vi "S4GUI.vi"(7 "Tab ObsEng":enum32{"Obs", "CCD modes", "Guider", "Eng"}(tab)) -> ()   [LabVIEW 2018] (continued)
            n2447 = call-dynamic "Read Stream.vi"("error in (no error)"=w4925, "Server in"=w4926) -> ("error out"=w4929:errorcluster, "Stream.lvclass"=w4932:refnum<class "Stream.lvclass">, "Server out"=w4930:refnum<class "Acquisition.lvclass">)  [unwired: 7 in]
            n2448 = disable-structure shown="Enabled" {
              disable-tunnel: w4932 -> [w4938 w4948]
              disable-tunnel: [w4937 w4948] -> w4931
              disable-tunnel: w4929 -> [w4935 w4947]
              disable-tunnel: [w4933 w4947] -> w4928
              frame Disabled {
                w4946 = FALSE ("Wait Until Done")
                n2449 = call-dynamic "Read comfile name1.vi"("error in (no error)"=w4935, "Stream in"=w4938) -> ("error out"=w4934:errorcluster, "comfile name1"=w4941:string, "Stream out"=w4936:refnum<class "Stream.lvclass">)  [unwired: 7 in]
                n2450 = call <vilib>:"Application Directory.vi"() -> ("Application Directory"=w4943:path)
                n2451 = Build Path(base path=w4943, name or relative path=w4941) -> (appended path=w4942:path)
                n2452 = Open VI Reference(vi path=w4942, error in (no error)=w4934) -> (vi reference=w4944:refnum<vi>, error out=w4945:errorcluster)  [unwired: 4 in]
                n2453 = invoke class="VI" method="Run VI"(reference=w4944, error in=w4945, "Wait until done"=w4946, "Auto Dispose Ref"=w4946) -> (reference out=w4940:refnum<vi>, error out=w4939:errorcluster)  [unwired: 1 in, 3 out]
                n2454 = call-dynamic "Write commfile ref1.vi"("error in (no error)"=w4939, "commfile ref1"=w4940, "Stream in"=w4936) -> ("error out"=w4933:errorcluster, "Stream out"=w4937:refnum<class "Stream.lvclass">)  [unwired: 7 in]
              }
              frame Enabled {
              }
            }
          }
        }
        n2455 = call-dynamic "Write Stream.vi"("error in (no error)"=w4898, "Stream.lvclass"=w4899, "Server in"=w4894) -> ("error out"=w4880:errorcluster, "Server out"=w4881:refnum<class "Acquisition.lvclass">)  [unwired: 7 in]
        n2456 = call-dynamic "Write enabled.vi"("error in (no error)"=w4880, "enabled"=w4877, "Server in"=w4881) -> ("error out"=w4878:errorcluster, "Server out"=w4879:refnum<class "Acquisition.lvclass">)  [unwired: 7 in]
        n2457 = call-dynamic "Write Channel.vi"("error in (no error)"=w4878, "Channel.lvclass"=w4882, "Acquisition in"=w4879) -> ("error out"=w4888:errorcluster, "Acquisition out"=w4887:refnum<class "Acquisition.lvclass">)  [unwired: 7 in]
        n2458 = call-dynamic "Write AcquisitionC.vi"("error in (no error)"=w4888, "Acquisition.lvclass"=w4887, "S4ACS_GUI in"=w4886) -> ("error out"=w4891:errorcluster, "S4ACS_GUI out"=w4892:refnum<class "S4GUI.lvclass">)  [unwired: 7 in]
      }
      event "CH4 on": Value Change {
        n2459 = event-data() -> ("NewVal"=w4954:bool)  [unwired: 1 in]
        n2460 = call-dynamic "Read AcquisitionD.vi"("error in (no error)"=w4972, "S4ACS_GUI in"=w4973) -> ("error out"=w4964:errorcluster, "Acquisition.lvclass"=w4969:refnum<class "Acquisition.lvclass">, "S4ACS_GUI out"=w4965:refnum<class "S4GUI.lvclass">)  [unwired: 7 in]
        n2461 = call-dynamic "Read Channel.vi"("error in (no error)"=w4964, "Acquisition in"=w4969) -> ("error out"=w4963:errorcluster, "Channel.lvclass"=w4958:refnum<class "Channel.lvclass">, "Acquisition out"=w4968:refnum<class "Acquisition.lvclass">)  [unwired: 7 in]
        n2462 = call-dynamic "Read Stream.vi"("error in (no error)"=w4963, "Server in"=w4968) -> ("error out"=w4956:errorcluster, "Stream.lvclass"=w4955:refnum<class "Stream.lvclass">, "Server out"=w4957:refnum<class "Acquisition.lvclass">)  [unwired: 7 in]
        n2463 = case shown="False" w4954 {
          selector: w4954 -> [w4974 w4996]
          tunnel: [w4980 w5000] -> w4950
          tunnel: w4955 -> [w4989 _]
          tunnel: [w4988 w5003] -> w4951
          tunnel: w4956 -> [w4975 w4997]
          tunnel: w4957 -> [w4976 w4998]
          tunnel: [w4976 w5002] -> w4952
          tunnel: w4958 -> [w4987 w4999]
          tunnel: [w4985 w4999] -> w4953
          tunnel: [w4974 w4996] -> w4949
          frame False {
            # "força FALSE nos parametros do CCD"
            n2464 = call-dynamic "Read Interface.vi"("error in (no error)"=w4975, "Channel in"=w4987) -> ("error out"=w4984:errorcluster, "Interface.lvclass"=w4978:refnum<class "Interface.lvclass">, "Channel out"=w4986:refnum<class "Channel.lvclass">)  [unwired: 7 in]
            n2465 = disable-structure shown="Disabled" {
              disable-tunnel: w4989 -> [w4993 w4995]
              disable-tunnel: [w4992 w4995] -> w4988
              disable-tunnel: [w4991 w4994] -> w4981
              disable-tunnel: w4975 -> [w4990 w4994]
              frame Disabled {
                n2466 = call-dynamic "End.vi"("error in (no error)"=w4990, "Stream in"=w4993) -> ("error out"=w4991:errorcluster, "Stream out"=w4992:refnum<class "Stream.lvclass">)  [unwired: 8 in]
              }
              frame Enabled {
              }
            }
            n2467 = call "Write Checked Params.vi"("error in (no error)"=w4984, "Checked Params"=T14 {"ACQUISITION_MODE"=FALSE, "TRIGGER_MODE"=FALSE, "READ_MODE"=FALSE, "PREAMP"=FALSE, "READOUT_RATE"=FALSE, "VERTICAL_SHIFT_SPEED"=FALSE, "EM_MODE"=FALSE, "EM_GAIN"=FALSE, "SHUTTER_MODE"=FALSE, "SHUTTER_TTL"=FALSE, "SHUTTER_OPENING_TIME"=FALSE, "SHUTTER_CLOSING_TIME"=FALSE, "VBIN"=FALSE, "HBIN"=FALSE, "INITIAL_LINE"=FALSE, "INITIAL_COLUMN"=FALSE, "FINAL_LINE"=FALSE, "FINAL_COLUMN"=FALSE, "FRAME_TRANSFER"=FALSE, "VERTICAL_CLOCK_VOLTAGE"=FALSE, "AD_CHANNEL"=FALSE}, "Interface in"=w4978) -> ("error out"=w4983:errorcluster, "Interface out"=w4977:refnum<class "Interface.lvclass">)  [unwired: 7 in]
            n2468 = call-dynamic "Write Interface.vi"("error in (no error)"=w4983, "Interface.lvclass"=w4977, "Channel in"=w4986) -> ("error out"=w4982:errorcluster, "Channel out"=w4985:refnum<class "Channel.lvclass">)  [unwired: 7 in]
            n2469 = Merge Errors(w4982, w4981) -> (w4980:errorcluster)
          }
          frame True {
            n2470 = call-dynamic "Read Stream.vi"("error in (no error)"=w4997, "Server in"=w4998) -> ("error out"=w5001:errorcluster, "Stream.lvclass"=w5004:refnum<class "Stream.lvclass">, "Server out"=w5002:refnum<class "Acquisition.lvclass">)  [unwired: 7 in]
            n2471 = disable-structure shown="Enabled" {
              disable-tunnel: w5004 -> [w5010 w5020]
              disable-tunnel: [w5009 w5020] -> w5003
              disable-tunnel: w5001 -> [w5007 w5019]
              disable-tunnel: [w5005 w5019] -> w5000
              frame Disabled {
                w5018 = FALSE ("Wait Until Done")
                n2472 = call-dynamic "Read comfile name1.vi"("error in (no error)"=w5007, "Stream in"=w5010) -> ("error out"=w5006:errorcluster, "comfile name1"=w5013:string, "Stream out"=w5008:refnum<class "Stream.lvclass">)  [unwired: 7 in]
                n2473 = call <vilib>:"Application Directory.vi"() -> ("Application Directory"=w5015:path)
                n2474 = Build Path(base path=w5015, name or relative path=w5013) -> (appended path=w5014:path)
                n2475 = Open VI Reference(vi path=w5014, error in (no error)=w5006) -> (vi reference=w5016:refnum<vi>, error out=w5017:errorcluster)  [unwired: 4 in]
                n2476 = invoke class="VI" method="Run VI"(reference=w5016, error in=w5017, "Wait until done"=w5018, "Auto Dispose Ref"=w5018) -> (reference out=w5012:refnum<vi>, error out=w5011:errorcluster)  [unwired: 1 in, 3 out]
                n2477 = call-dynamic "Write commfile ref1.vi"("error in (no error)"=w5011, "commfile ref1"=w5012, "Stream in"=w5008) -> ("error out"=w5005:errorcluster, "Stream out"=w5009:refnum<class "Stream.lvclass">)  [unwired: 7 in]
              }
              frame Enabled {
              }
            }
          }
        }
        n2478 = call-dynamic "Write Stream.vi"("error in (no error)"=w4950, "Stream.lvclass"=w4951, "Server in"=w4952) -> ("error out"=w4960:errorcluster, "Server out"=w4962:refnum<class "Acquisition.lvclass">)  [unwired: 7 in]
        n2479 = call-dynamic "Write enabled.vi"("error in (no error)"=w4960, "enabled"=w4949, "Server in"=w4962) -> ("error out"=w4959:errorcluster, "Server out"=w4961:refnum<class "Acquisition.lvclass">)  [unwired: 7 in]
        n2480 = call-dynamic "Write Channel.vi"("error in (no error)"=w4959, "Channel.lvclass"=w4953, "Acquisition in"=w4961) -> ("error out"=w4967:errorcluster, "Acquisition out"=w4966:refnum<class "Acquisition.lvclass">)  [unwired: 7 in]
        n2481 = call-dynamic "Write AcquisitionD.vi"("error in (no error)"=w4967, "Acquisition.lvclass"=w4966, "S4ACS_GUI in"=w4965) -> ("error out"=w4970:errorcluster, "S4ACS_GUI out"=w4971:refnum<class "S4GUI.lvclass">)  [unwired: 7 in]
      }
      event "Run WPROT": Value Change {
        n2482 = event-data() -> ("NewVal"=w5028:bool)  [unwired: 1 in]
        n2483 = case shown="True" w5028 {
          tunnel: [u32 0 ("Ciclos  WPROT") "Ciclos  WPROT"] -> w5027
          tunnel: w5024 -> [w5030 w5035]
          tunnel: [w5030 w5034] -> w5023
          tunnel: w5022 -> [w5029 w5033]
          tunnel: [w5029 w5032] -> w5021
          frame False {
          }
          frame True {
            n2484 = call-dynamic "Write Obs_state.vi"("error in (no error)"=w5033, "Obs_state"=u32 350, "S4ACS_GUI in"=w5035) -> ("error out"=w5032:errorcluster, "S4ACS_GUI out"=w5034:refnum<class "S4GUI.lvclass">)  [unwired: 7 in]
          }
        }
        n2485 = call-dynamic "Write cycles wprot.vi"("error in (no error)"=w5021, "cycles wprot"=w5027, "S4GUI in"=w5023) -> ("error out"=w5025:errorcluster, "S4GUI out"=w5026:refnum<class "S4GUI.lvclass">)  [unwired: 7 in]
      }
      event "Start SM": Value Change {
        n2486 = event-data() -> ()  [unwired: 1 in, 6 out]
        n2487 = call-dynamic "Read Obs_state.vi"("error in (no error)"=w5064, "S4ACS_GUI in"=w5065) -> ("error out"=w5051:errorcluster, "Obs_state"=w5062:u32, "S4ACS_GUI out"=w5053:refnum<class "S4GUI.lvclass">)  [unwired: 7 in]
        n2488 = call "Read Instrument.lvclass.vi"("error in (no error)"=w5051, "S4ACS_GUI in"=w5053) -> ("error out"=w5049:errorcluster, "Instrument.lvclass"=w5050:refnum<class "Instrument.lvclass">, "S4ACS_GUI out"=w5052:refnum<class "S4GUI.lvclass">)  [unwired: 7 in]
        n2489 = Not Equal?(x=w5062, y=u32 400) -> (x != y?=w5061:bool)
        n2490 = call-dynamic "Read mode.vi"("error in (no error)"=w5049, "Instrument in"=w5050) -> ("error out"=w5048:errorcluster, "mode"=w5047:bool)  [unwired: 7 in, 1 out]
        n2491 = case shown="True" w5061 {
          tunnel: w5052 -> [w5107 w5195]
          tunnel: w5048 -> [w5108 w5194]
          tunnel: [w5111 w5201] -> w5042
          tunnel: [w5110 w5202] -> w5041
          tunnel: w5058 -> [_ w5209]
          tunnel: w5057 -> [_ w5208]
          tunnel: w5056 -> [_ w5207]
          tunnel: w5055 -> [_ w5206]
          tunnel: w5054 -> [_ w5205]
          tunnel: w5047 -> [_ w5204]
          tunnel: w5046 -> [_ w5185]
          tunnel: w5045 -> [_ w5188]
          tunnel: w5044 -> [_ w5187]
          tunnel: w5043 -> [_ w5186]
          tunnel: ["RESUME SM CLICKED" ("User Event") "START SM" ("User Event")] -> w5038
          frame False {
            # "Obs_state=400 (PAUSED), envia RESUME e vai para Obs_state=500 \npara esperar envio do comando RESUME a todos os canais."
            n2492 = call-dynamic "Write Obs_state.vi"("error in (no error)"=w5108, "Obs_state"=500, "S4ACS_GUI in"=w5107) -> ("error out"=w5112:errorcluster, "S4ACS_GUI out"=w5113:refnum<class "S4GUI.lvclass">)  [unwired: 7 in]
            n2493 = call-dynamic "Read AcquisitionA.vi"("error in (no error)"=w5112, "S4ACS_GUI in"=w5113) -> ("error out"=w5099:errorcluster, "Acquisition.lvclass"=w5103:refnum<class "Acquisition.lvclass">, "S4ACS_GUI out"=w5123:refnum<class "S4GUI.lvclass">)  [unwired: 7 in]
            n2494 = call-dynamic "Read enabled.vi"("error in (no error)"=w5099, "Server in"=w5103) -> ("error out"=w5101:errorcluster, "enabled"=w5100:bool, "Server out"=w5102:refnum<class "Acquisition.lvclass">)  [unwired: 7 in]
            n2495 = call-dynamic "Read Channel.vi"("error in (no error)"=w5101, "Acquisition in"=w5102) -> ("error out"=w5104:errorcluster, "Channel.lvclass"=w5105:refnum<class "Channel.lvclass">, "Acquisition out"=w5122:refnum<class "Acquisition.lvclass">)  [unwired: 7 in]
            n2496 = case shown="True" w5100 {
              tunnel: w5122 -> [w5170 w5183]
              tunnel: [w5170 w5182] -> w5121
              tunnel: [w5169 w5179] -> w5120
              tunnel: w5105 -> [_ w5172]
              tunnel: w5104 -> [w5169 w5171]
              frame False {
              }
              frame True {
                n2497 = call-dynamic "Read State Machine.vi"("error in (no error)"=w5171, "Device in"=w5172) -> ("error out"=w5173:errorcluster, "State Machine.lvclass"=w5174:refnum<class "State Machine.lvclass">, "Device out"=w5178:refnum<class "Channel.lvclass">)  [unwired: 7 in]
                n2498 = call "Next State.vi"("error in (no error)"=w5173, "New_State"=96, "State Machine in"=w5174) -> ("error out"=w5175:errorcluster, "State Machine out"=w5177:refnum<class "State Machine.lvclass">)  [unwired: 7 in]
                n2499 = call-dynamic "Write State Machine.vi"("error in (no error)"=w5175, "State Machine.lvclass"=w5177, "Device in"=w5178) -> ("error out"=w5180:errorcluster, "Device out"=w5181:refnum<class "Channel.lvclass">)  [unwired: 7 in]
                n2500 = call-dynamic "Write Channel.vi"("error in (no error)"=w5180, "Channel.lvclass"=w5181, "Acquisition in"=w5183) -> ("error out"=w5179:errorcluster, "Acquisition out"=w5182:refnum<class "Acquisition.lvclass">)  [unwired: 7 in]
              }
            }
            n2501 = call-dynamic "Write AcquisitionA.vi"("error in (no error)"=w5120, "Acquisition.lvclass"=w5121, "S4ACS_GUI in"=w5123) -> ("error out"=w5119:errorcluster, "S4ACS_GUI out"=w5116:refnum<class "S4GUI.lvclass">)  [unwired: 7 in]
            n2502 = call "Read AcquisitionB.vi"("error in (no error)"=w5119, "S4ACS_GUI in"=w5116) -> ("error out"=w5090:errorcluster, "Acquisition.lvclass"=w5091:refnum<class "Acquisition.lvclass">, "S4ACS_GUI out"=w5092:refnum<class "S4GUI.lvclass">)  [unwired: 7 in]
            n2503 = call-dynamic "Read enabled.vi"("error in (no error)"=w5090, "Server in"=w5091) -> ("error out"=w5094:errorcluster, "enabled"=w5093:bool, "Server out"=w5095:refnum<class "Acquisition.lvclass">)  [unwired: 7 in]
            n2504 = call-dynamic "Read Channel.vi"("error in (no error)"=w5094, "Acquisition in"=w5095) -> ("error out"=w5096:errorcluster, "Channel.lvclass"=w5097:refnum<class "Channel.lvclass">, "Acquisition out"=w5098:refnum<class "Acquisition.lvclass">)  [unwired: 7 in]
            n2505 = case shown="True" w5093 {
              tunnel: w5098 -> [w5155 w5168]
              tunnel: [w5155 w5167] -> w5089
              tunnel: [w5154 w5164] -> w5088
              tunnel: w5097 -> [_ w5157]
              tunnel: w5096 -> [w5154 w5156]
              frame False {
              }
              frame True {
                n2506 = call-dynamic "Read State Machine.vi"("error in (no error)"=w5156, "Device in"=w5157) -> ("error out"=w5158:errorcluster, "State Machine.lvclass"=w5159:refnum<class "State Machine.lvclass">, "Device out"=w5163:refnum<class "Channel.lvclass">)  [unwired: 7 in]
                n2507 = call "Next State.vi"("error in (no error)"=w5158, "New_State"=96, "State Machine in"=w5159) -> ("error out"=w5160:errorcluster, "State Machine out"=w5162:refnum<class "State Machine.lvclass">)  [unwired: 7 in]
                n2508 = call-dynamic "Write State Machine.vi"("error in (no error)"=w5160, "State Machine.lvclass"=w5162, "Device in"=w5163) -> ("error out"=w5165:errorcluster, "Device out"=w5166:refnum<class "Channel.lvclass">)  [unwired: 7 in]
                n2509 = call-dynamic "Write Channel.vi"("error in (no error)"=w5165, "Channel.lvclass"=w5166, "Acquisition in"=w5168) -> ("error out"=w5164:errorcluster, "Acquisition out"=w5167:refnum<class "Acquisition.lvclass">)  [unwired: 7 in]
              }
            }
            n2510 = call "Write AcquisitionB.vi"("error in (no error)"=w5088, "Acquisition.lvclass"=w5089, "S4ACS_GUI in"=w5092) -> ("error out"=w5118:errorcluster, "S4ACS_GUI out"=w5115:refnum<class "S4GUI.lvclass">)  [unwired: 7 in]
            n2511 = call-dynamic "Read AcquisitionC.vi"("error in (no error)"=w5118, "S4ACS_GUI in"=w5115) -> ("error out"=w5078:errorcluster, "Acquisition.lvclass"=w5081:refnum<class "Acquisition.lvclass">, "S4ACS_GUI out"=w5080:refnum<class "S4GUI.lvclass">)  [unwired: 7 in]
            n2512 = call-dynamic "Read enabled.vi"("error in (no error)"=w5078, "Server in"=w5081) -> ("error out"=w5083:errorcluster, "enabled"=w5082:bool, "Server out"=w5084:refnum<class "Acquisition.lvclass">)  [unwired: 7 in]
            n2513 = call-dynamic "Read Channel.vi"("error in (no error)"=w5083, "Acquisition in"=w5084) -> ("error out"=w5085:errorcluster, "Channel.lvclass"=w5086:refnum<class "Channel.lvclass">, "Acquisition out"=w5087:refnum<class "Acquisition.lvclass">)  [unwired: 7 in]
            n2514 = case shown="True" w5082 {
              tunnel: w5087 -> [w5140 w5153]
              tunnel: [w5140 w5152] -> w5079
              tunnel: [w5139 w5149] -> w5077
              tunnel: w5086 -> [_ w5142]
              tunnel: w5085 -> [w5139 w5141]
              frame False {
              }
              frame True {
                n2515 = call-dynamic "Read State Machine.vi"("error in (no error)"=w5141, "Device in"=w5142) -> ("error out"=w5143:errorcluster, "State Machine.lvclass"=w5144:refnum<class "State Machine.lvclass">, "Device out"=w5148:refnum<class "Channel.lvclass">)  [unwired: 7 in]
                n2516 = call "Next State.vi"("error in (no error)"=w5143, "New_State"=96, "State Machine in"=w5144) -> ("error out"=w5145:errorcluster, "State Machine out"=w5147:refnum<class "State Machine.lvclass">)  [unwired: 7 in]
                n2517 = call-dynamic "Write State Machine.vi"("error in (no error)"=w5145, "State Machine.lvclass"=w5147, "Device in"=w5148) -> ("error out"=w5150:errorcluster, "Device out"=w5151:refnum<class "Channel.lvclass">)  [unwired: 7 in]
                n2518 = call-dynamic "Write Channel.vi"("error in (no error)"=w5150, "Channel.lvclass"=w5151, "Acquisition in"=w5153) -> ("error out"=w5149:errorcluster, "Acquisition out"=w5152:refnum<class "Acquisition.lvclass">)  [unwired: 7 in]
              }
            }
            n2519 = call-dynamic "Write AcquisitionC.vi"("error in (no error)"=w5077, "Acquisition.lvclass"=w5079, "S4ACS_GUI in"=w5080) -> ("error out"=w5117:errorcluster, "S4ACS_GUI out"=w5114:refnum<class "S4GUI.lvclass">)  [unwired: 7 in]
            n2520 = call-dynamic "Read AcquisitionD.vi"("error in (no error)"=w5117, "S4ACS_GUI in"=w5114) -> ("error out"=w5068:errorcluster, "Acquisition.lvclass"=w5069:refnum<class "Acquisition.lvclass">, "S4ACS_GUI out"=w5070:refnum<class "S4GUI.lvclass">)  [unwired: 7 in]
            n2521 = call-dynamic "Read enabled.vi"("error in (no error)"=w5068, "Server in"=w5069) -> ("error out"=w5072:errorcluster, "enabled"=w5071:bool, "Server out"=w5073:refnum<class "Acquisition.lvclass">)  [unwired: 7 in]
            n2522 = call-dynamic "Read Channel.vi"("error in (no error)"=w5072, "Acquisition in"=w5073) -> ("error out"=w5074:errorcluster, "Channel.lvclass"=w5075:refnum<class "Channel.lvclass">, "Acquisition out"=w5076:refnum<class "Acquisition.lvclass">)  [unwired: 7 in]
            n2523 = case shown="True" w5071 {
              tunnel: w5076 -> [w5125 w5138]
              tunnel: [w5125 w5137] -> w5067
              tunnel: [w5124 w5134] -> w5066
              tunnel: w5075 -> [_ w5127]
              tunnel: w5074 -> [w5124 w5126]
              frame False {
              }
              frame True {
                n2524 = call-dynamic "Read State Machine.vi"("error in (no error)"=w5126, "Device in"=w5127) -> ("error out"=w5128:errorcluster, "State Machine.lvclass"=w5129:refnum<class "State Machine.lvclass">, "Device out"=w5133:refnum<class "Channel.lvclass">)  [unwired: 7 in]
                n2525 = call "Next State.vi"("error in (no error)"=w5128, "New_State"=96, "State Machine in"=w5129) -> ("error out"=w5130:errorcluster, "State Machine out"=w5132:refnum<class "State Machine.lvclass">)  [unwired: 7 in]
                n2526 = call-dynamic "Write State Machine.vi"("error in (no error)"=w5130, "State Machine.lvclass"=w5132, "Device in"=w5133) -> ("error out"=w5135:errorcluster, "Device out"=w5136:refnum<class "Channel.lvclass">)  [unwired: 7 in]
                n2527 = call-dynamic "Write Channel.vi"("error in (no error)"=w5135, "Channel.lvclass"=w5136, "Acquisition in"=w5138) -> ("error out"=w5134:errorcluster, "Acquisition out"=w5137:refnum<class "Acquisition.lvclass">)  [unwired: 7 in]
              }
            }
            n2528 = call-dynamic "Write AcquisitionD.vi"("error in (no error)"=w5066, "Acquisition.lvclass"=w5067, "S4ACS_GUI in"=w5070) -> ("error out"=w5110:errorcluster, "S4ACS_GUI out"=w5111:refnum<class "S4GUI.lvclass">)  [unwired: 7 in]
          }
          frame True {
            # "vide S4GUI:\nHandleObservationSync.vi"
            # "aba atual em Tab Acq Type"
            n2529 = call "Read Instrument.lvclass.vi"("error in (no error)"=w5194, "S4ACS_GUI in"=w5195) -> ("error out"=w5197:errorcluster, "Instrument.lvclass"=w5199:refnum<class "Instrument.lvclass">, "S4ACS_GUI out"=w5192:refnum<class "S4GUI.lvclass">)  [unwired: 7 in]
            n2530 = call "Read WPROT.vi"("error in (no error)"=w5197, "Instrument in"=w5199) -> ("error out"=w5196:errorcluster, "Opt_Selector.lvclass"=w5198:refnum<class "Opt_Selector.lvclass">)  [unwired: 7 in, 1 out]
            n2531 = call-dynamic "Read sequencia.vi"("error in (no error)"=w5196, "Opt_Selector in"=w5198) -> ("error out"=w5191:errorcluster, "sequencia"=w5193:u16)  [unwired: 7 in, 1 out]
            n2532 = case shown="\"FOCUS\"" w5185 {
              tunnel: [u32 271 ("Obs_state") u32 251 ("Obs_state")] -> w5212
              tunnel: w5192 -> [w5233 w5236]
              tunnel: w5191 -> [w5223 w5235]
              tunnel: [w5231 w5236] -> w5190
              tunnel: [w5222 w5235] -> w5189
              tunnel: w5188 -> [w5230 _]
              tunnel: w5187 -> [w5229 _]
              tunnel: w5186 -> [w5228 _]
              frame "FOCUS" {
                n2533 = call-dynamic "Read TelFocus.lvclass.vi"("error in (no error)"=w5223, "S4GUI in"=w5233) -> ("error out"=w5225:errorcluster, "TelFocus.lvclass"=w5227:refnum<class "TelFocus.lvclass">, "S4GUI out"=w5232:refnum<class "S4GUI.lvclass">)  [unwired: 7 in]
                n2534 = call-dynamic "LoadParam.vi"("#steps"=w5228, "error in (no error)"=w5225, "step"=w5229, "init"=w5230, "TelFocus in"=w5227) -> ("error out"=w5224:errorcluster, "TelFocus out"=w5226:refnum<class "TelFocus.lvclass">)  [unwired: 5 in]
                n2535 = call-dynamic "Write TelFocus.lvclass.vi"("error in (no error)"=w5224, "TelFocus.lvclass"=w5226, "S4GUI in"=w5232) -> ("error out"=w5222:errorcluster, "S4GUI out"=w5231:refnum<class "S4GUI.lvclass">)  [unwired: 7 in]
              }
              frame Default {
              }
            }
            n2536 = case shown="Default" w5185 {
              tunnel: w5204 -> [_ w5218]
              tunnel: [u32 1 ("# Cycles") w5217] -> w5203
              tunnel: [u32 1 w5216] -> w5200
              tunnel: w5193 -> [_ w5215]
              frame "FOCUS" {
                # "Aba FOCUS: Para a sequencia de foco, sempre  #Cycles=1 e #Seqs=1"
              }
              frame Default {
                n2537 = case shown="False" w5218 {
                  tunnel: [0 w5221] -> w5216
                  tunnel: w5215 -> [_ w5220]
                  frame False {
                    # "OV 20230424: \n#SEQ agora armazena as\nposições da lâmina utilizadas.\nNa fotometria, #SEQ=0"
                    # "fotometria:"
                  }
                  frame True {
                    # "OV 20230424: \n#SEQ agora armazena as\nposições da lâmina utilizadas.\nNa polarimetria, #SEQ=WPROT.sequencia"
                    # "polarimetria:"
                    n2538 = To Unsigned Long Integer(number=w5220) -> (unsigned 32bit integer=w5221:u32)
                  }
                }
                n2539 = local read "# Cycles"() -> (w5217:u32)
              }
            }
            n2540 = call-dynamic "Write Obs_state.vi"("error in (no error)"=w5189, "Obs_state"=w5212, "S4ACS_GUI in"=w5190) -> ("error out"=w5211:errorcluster, "S4ACS_GUI out"=w5210:refnum<class "S4GUI.lvclass">)  [unwired: 7 in]
            n2541 = stacked-sequence {
              seq-local: [w5260 _ _ _] -> [_ w5332 _ _]
              seq-local: [w5259 _ _ _] -> [_ w5331 _ _]
              seq-local: [_ w5330 _ _] -> [_ _ w5383 _]
              seq-local: [_ w5329 _ _] -> [_ _ w5382 _]
              seq-local: [_ _ w5381 _] -> [_ _ _ w5434]
              seq-local: [_ _ w5380 _] -> [_ _ _ w5433]
              tunnel: w5211 -> [w5275 _ _ _]
              tunnel: w5210 -> [w5274 _ _ _]
              tunnel: [_ _ _ w5432] -> w5201
              tunnel: [_ _ _ w5431] -> w5202
              tunnel: w5209 -> [w5258 w5328 w5379 w5430]
              tunnel: w5208 -> [w5257 w5327 w5359 w5410]
              tunnel: w5207 -> [w5256 w5307 w5358 w5409]
              tunnel: w5206 -> [w5255 w5306 w5357 w5408]
              tunnel: w5205 -> [w5250 w5303 w5354 w5405]
              tunnel: w5203 -> [_ _ _ _]
              tunnel: w5200 -> [_ _ _ _]
              tunnel: w5185 -> [w5242 w5297 w5348 w5397]
              frame #0 {
                # "object"
                # "suffix"
                # "obsType"
                n2542 = local read "Exptime ch1"() -> (w5243:dbl)
                n2543 = call-dynamic "Read AcquisitionA.vi"("error in (no error)"=w5275, "S4ACS_GUI in"=w5274) -> ("error out"=w5273:errorcluster, "Acquisition.lvclass"=w5272:refnum<class "Acquisition.lvclass">, "S4ACS_GUI out"=w5263:refnum<class "S4GUI.lvclass">)  [unwired: 7 in]
                n2544 = call-dynamic "Read Channel.vi"("error in (no error)"=w5273, "Acquisition in"=w5272) -> ("error out"=w5270:errorcluster, "Channel.lvclass"=w5271:refnum<class "Channel.lvclass">, "Acquisition out"=w5262:refnum<class "Acquisition.lvclass">)  [unwired: 7 in]
                n2545 = call-dynamic "Read Interface.vi"("error in (no error)"=w5270, "Channel in"=w5271) -> ("error out"=w5281:errorcluster, "Interface.lvclass"=w5268:refnum<class "Interface.lvclass">, "Channel out"=w5269:refnum<class "Channel.lvclass">)  [unwired: 7 in]
                n2546 = call "Write Exposure Time.vi"("error in (no error)"=w5281, "Exposure Time"=w5243, "Interface in"=w5268) -> ("error out"=w5244:errorcluster, "Interface out"=w5247:refnum<class "Interface.lvclass">)  [unwired: 7 in]
                n2547 = case shown="Default" w5242 {
                  tunnel: w5247 -> [w5283 w5288]
                  tunnel: [w5283 w5287] -> w5246
                  tunnel: [w5282 w5286] -> w5245
                  tunnel: w5244 -> [w5282 w5285]
                  tunnel: w5243 -> [_ w5284]
                  frame "ZERO" {
                  }
                  frame Default {
                    n2548 = call-dynamic "Write prev ExpTime.vi"("error in (no error)"=w5285, "prev ExpTime"=w5284, "Interface in"=w5288) -> ("error out"=w5286:errorcluster, "Interface out"=w5287:refnum<class "Interface.lvclass">)  [unwired: 7 in]
                  }
                }
                n2549 = call-dynamic "Write Suffix.vi"("error in (no error)"=w5245, "Suffix"=w5258, "Interface in"=w5246) -> ("error out"=w5280:errorcluster, "Interface out"=w5267:refnum<class "Interface.lvclass">)  [unwired: 7 in]
                n2550 = call-dynamic "Write ObsType.vi"("error in (no error)"=w5280, "ObsType"=w5256, "Interface in"=w5267) -> ("error out"=w5279:errorcluster, "Interface out"=w5266:refnum<class "Interface.lvclass">)  [unwired: 7 in]
                n2551 = call-dynamic "Write Object.vi"("error in (no error)"=w5279, "Object"=w5255, "Interface in"=w5266) -> ("error out"=w5278:errorcluster, "Interface out"=w5265:refnum<class "Interface.lvclass">)  [unwired: 7 in]
                n2552 = call-dynamic "Write Comments.vi"("error in (no error)"=w5278, "Comments"=w5257, "Interface in"=w5265) -> ("error out"=w5277:errorcluster, "Interface out"=w5264:refnum<class "Interface.lvclass">)  [unwired: 7 in]
                n2553 = call-dynamic "Write DS9.vi"("error in (no error)"=w5277, "DS9"="F", "Interface in"=w5264) -> ("error out"=w5252:errorcluster, "Interface out"=w5254:refnum<class "Interface.lvclass">)  [unwired: 7 in]
                n2554 = call-dynamic "Write Observer.vi"("error in (no error)"=w5252, "Observer"=w5250, "Interface in"=w5254) -> ("error out"=w5251:errorcluster, "Interface out"=w5253:refnum<class "Interface.lvclass">)  [unwired: 7 in]
                n2555 = property on="Exposure Time ch1" class="Slide (strict)"("Scale.Maximum"=w5243, "Scale.Minimum"=0.0 ("Scale.Range:Minimum")) -> ()  [unwired: 2 in, 2 out]
                n2556 = call-dynamic "Write Interface.vi"("error in (no error)"=w5251, "Interface.lvclass"=w5253, "Channel in"=w5269) -> ("error out"=w5249:errorcluster, "Channel out"=w5248:refnum<class "Channel.lvclass">)  [unwired: 7 in]
                n2557 = call-dynamic "Write Channel.vi"("error in (no error)"=w5249, "Channel.lvclass"=w5248, "Acquisition in"=w5262) -> ("error out"=w5239:errorcluster, "Acquisition out"=w5241:refnum<class "Acquisition.lvclass">)  [unwired: 7 in]
                n2558 = call-dynamic "CalcCubeDuration.vi"("error in (no error)"=w5239, "Acquisition in"=w5241) -> ("error out"=w5238:errorcluster, "Acquisition out"=w5240:refnum<class "Acquisition.lvclass">)  [unwired: 8 in]
                n2559 = call-dynamic "Write AcquisitionA.vi"("error in (no error)"=w5238, "Acquisition.lvclass"=w5240, "S4ACS_GUI in"=w5263) -> ("error out"=w5259:errorcluster, "S4ACS_GUI out"=w5260:refnum<class "S4GUI.lvclass">)  [unwired: 7 in]
              }
              frame #1 {
                # "object"
                # "suffix"
                # "obsType"
                n2560 = call "Read AcquisitionB.vi"("error in (no error)"=w5331, "S4ACS_GUI in"=w5332) -> ("error out"=w5315:errorcluster, "Acquisition.lvclass"=w5316:refnum<class "Acquisition.lvclass">, "S4ACS_GUI out"=w5325:refnum<class "S4GUI.lvclass">)  [unwired: 7 in]
                n2561 = local read "Exptime ch2"() -> (w5298:dbl)
                n2562 = call-dynamic "Read Channel.vi"("error in (no error)"=w5315, "Acquisition in"=w5316) -> ("error out"=w5318:errorcluster, "Channel.lvclass"=w5317:refnum<class "Channel.lvclass">, "Acquisition out"=w5326:refnum<class "Acquisition.lvclass">)  [unwired: 7 in]
                n2563 = call-dynamic "Read Interface.vi"("error in (no error)"=w5318, "Channel in"=w5317) -> ("error out"=w5310:errorcluster, "Interface.lvclass"=w5320:refnum<class "Interface.lvclass">, "Channel out"=w5319:refnum<class "Channel.lvclass">)  [unwired: 7 in]
                n2564 = call "Write Exposure Time.vi"("error in (no error)"=w5310, "Exposure Time"=w5298, "Interface in"=w5320) -> ("error out"=w5299:errorcluster, "Interface out"=w5300:refnum<class "Interface.lvclass">)  [unwired: 7 in]
                n2565 = case shown="Default" w5297 {
                  tunnel: w5300 -> [w5334 w5339]
                  tunnel: [w5334 w5338] -> w5296
                  tunnel: [w5333 w5337] -> w5295
                  tunnel: w5299 -> [w5333 w5336]
                  tunnel: w5298 -> [_ w5335]
                  frame "ZERO" {
                  }
                  frame Default {
                    n2566 = call-dynamic "Write prev ExpTime.vi"("error in (no error)"=w5336, "prev ExpTime"=w5335, "Interface in"=w5339) -> ("error out"=w5337:errorcluster, "Interface out"=w5338:refnum<class "Interface.lvclass">)  [unwired: 7 in]
                  }
                }
                n2567 = call-dynamic "Write Suffix.vi"("error in (no error)"=w5295, "Suffix"=w5328, "Interface in"=w5296) -> ("error out"=w5311:errorcluster, "Interface out"=w5321:refnum<class "Interface.lvclass">)  [unwired: 7 in]
                n2568 = call-dynamic "Write ObsType.vi"("error in (no error)"=w5311, "ObsType"=w5307, "Interface in"=w5321) -> ("error out"=w5312:errorcluster, "Interface out"=w5322:refnum<class "Interface.lvclass">)  [unwired: 7 in]
                n2569 = call-dynamic "Write Object.vi"("error in (no error)"=w5312, "Object"=w5306, "Interface in"=w5322) -> ("error out"=w5313:errorcluster, "Interface out"=w5323:refnum<class "Interface.lvclass">)  [unwired: 7 in]
                n2570 = call-dynamic "Write Comments.vi"("error in (no error)"=w5313, "Comments"=w5327, "Interface in"=w5323) -> ("error out"=w5314:errorcluster, "Interface out"=w5324:refnum<class "Interface.lvclass">)  [unwired: 7 in]
                n2571 = call-dynamic "Write DS9.vi"("error in (no error)"=w5314, "DS9"="F", "Interface in"=w5324) -> ("error out"=w5304:errorcluster, "Interface out"=w5305:refnum<class "Interface.lvclass">)  [unwired: 7 in]
                n2572 = call-dynamic "Write Observer.vi"("error in (no error)"=w5304, "Observer"=w5303, "Interface in"=w5305) -> ("error out"=w5289:errorcluster, "Interface out"=w5290:refnum<class "Interface.lvclass">)  [unwired: 7 in]
                n2573 = property on="Exposure Time ch2" class="Slide (strict)"("Scale.Maximum"=w5298, "Scale.Minimum"=0.0 ("Scale.Range:Minimum")) -> ()  [unwired: 2 in, 2 out]
                n2574 = call-dynamic "Write Interface.vi"("error in (no error)"=w5289, "Interface.lvclass"=w5290, "Channel in"=w5319) -> ("error out"=w5302:errorcluster, "Channel out"=w5301:refnum<class "Channel.lvclass">)  [unwired: 7 in]
                n2575 = call-dynamic "Write Channel.vi"("error in (no error)"=w5302, "Channel.lvclass"=w5301, "Acquisition in"=w5326) -> ("error out"=w5292:errorcluster, "Acquisition out"=w5294:refnum<class "Acquisition.lvclass">)  [unwired: 7 in]
                n2576 = call-dynamic "CalcCubeDuration.vi"("error in (no error)"=w5292, "Acquisition in"=w5294) -> ("error out"=w5291:errorcluster, "Acquisition out"=w5293:refnum<class "Acquisition.lvclass">)  [unwired: 8 in]
                n2577 = call "Write AcquisitionB.vi"("error in (no error)"=w5291, "Acquisition.lvclass"=w5293, "S4ACS_GUI in"=w5325) -> ("error out"=w5329:errorcluster, "S4ACS_GUI out"=w5330:refnum<class "S4GUI.lvclass">)  [unwired: 7 in]
              }
              frame #2 {
                # "object"
                # "suffix"
                # "obsType"
                n2578 = call-dynamic "Read AcquisitionC.vi"("error in (no error)"=w5382, "S4ACS_GUI in"=w5383) -> ("error out"=w5373:errorcluster, "Acquisition.lvclass"=w5372:refnum<class "Acquisition.lvclass">, "S4ACS_GUI out"=w5363:refnum<class "S4GUI.lvclass">)  [unwired: 7 in]
                n2579 = call-dynamic "Read Channel.vi"("error in (no error)"=w5373, "Acquisition in"=w5372) -> ("error out"=w5370:errorcluster, "Channel.lvclass"=w5371:refnum<class "Channel.lvclass">, "Acquisition out"=w5362:refnum<class "Acquisition.lvclass">)  [unwired: 7 in]
                n2580 = local read "Exptime ch3"() -> (w5349:dbl)
                n2581 = call-dynamic "Read Interface.vi"("error in (no error)"=w5370, "Channel in"=w5371) -> ("error out"=w5378:errorcluster, "Interface.lvclass"=w5368:refnum<class "Interface.lvclass">, "Channel out"=w5369:refnum<class "Channel.lvclass">)  [unwired: 7 in]
                n2582 = call "Write Exposure Time.vi"("error in (no error)"=w5378, "Exposure Time"=w5349, "Interface in"=w5368) -> ("error out"=w5350:errorcluster, "Interface out"=w5351:refnum<class "Interface.lvclass">)  [unwired: 7 in]
                n2583 = case shown="\"ZERO\"" w5348 {
                  tunnel: w5351 -> [w5385 w5390]
                  tunnel: [w5385 w5389] -> w5347
                  tunnel: [w5384 w5388] -> w5346
                  tunnel: w5350 -> [w5384 w5387]
                  tunnel: w5349 -> [_ w5386]
                  frame "ZERO" {
                  }
                  frame Default {
                    n2584 = call-dynamic "Write prev ExpTime.vi"("error in (no error)"=w5387, "prev ExpTime"=w5386, "Interface in"=w5390) -> ("error out"=w5388:errorcluster, "Interface out"=w5389:refnum<class "Interface.lvclass">)  [unwired: 7 in]
                  }
                }
                n2585 = call-dynamic "Write Suffix.vi"("error in (no error)"=w5346, "Suffix"=w5379, "Interface in"=w5347) -> ("error out"=w5377:errorcluster, "Interface out"=w5367:refnum<class "Interface.lvclass">)  [unwired: 7 in]
                n2586 = call-dynamic "Write ObsType.vi"("error in (no error)"=w5377, "ObsType"=w5358, "Interface in"=w5367) -> ("error out"=w5376:errorcluster, "Interface out"=w5366:refnum<class "Interface.lvclass">)  [unwired: 7 in]
                n2587 = call-dynamic "Write Object.vi"("error in (no error)"=w5376, "Object"=w5357, "Interface in"=w5366) -> ("error out"=w5375:errorcluster, "Interface out"=w5365:refnum<class "Interface.lvclass">)  [unwired: 7 in]
                n2588 = call-dynamic "Write Comments.vi"("error in (no error)"=w5375, "Comments"=w5359, "Interface in"=w5365) -> ("error out"=w5374:errorcluster, "Interface out"=w5364:refnum<class "Interface.lvclass">)  [unwired: 7 in]
                n2589 = call-dynamic "Write DS9.vi"("error in (no error)"=w5374, "DS9"="F", "Interface in"=w5364) -> ("error out"=w5355:errorcluster, "Interface out"=w5356:refnum<class "Interface.lvclass">)  [unwired: 7 in]
                n2590 = property on="Exposure Time ch3" class="Slide (strict)"("Scale.Maximum"=w5349, "Scale.Minimum"=0.0 ("Scale.Range:Minimum")) -> ()  [unwired: 2 in, 2 out]
                n2591 = call-dynamic "Write Observer.vi"("error in (no error)"=w5355, "Observer"=w5354, "Interface in"=w5356) -> ("error out"=w5340:errorcluster, "Interface out"=w5341:refnum<class "Interface.lvclass">)  [unwired: 7 in]
                n2592 = call-dynamic "Write Interface.vi"("error in (no error)"=w5340, "Interface.lvclass"=w5341, "Channel in"=w5369) -> ("error out"=w5353:errorcluster, "Channel out"=w5352:refnum<class "Channel.lvclass">)  [unwired: 7 in]
                n2593 = call-dynamic "Write Channel.vi"("error in (no error)"=w5353, "Channel.lvclass"=w5352, "Acquisition in"=w5362) -> ("error out"=w5343:errorcluster, "Acquisition out"=w5345:refnum<class "Acquisition.lvclass">)  [unwired: 7 in]
                n2594 = call-dynamic "CalcCubeDuration.vi"("error in (no error)"=w5343, "Acquisition in"=w5345) -> ("error out"=w5342:errorcluster, "Acquisition out"=w5344:refnum<class "Acquisition.lvclass">)  [unwired: 8 in]
                n2595 = call-dynamic "Write AcquisitionC.vi"("error in (no error)"=w5342, "Acquisition.lvclass"=w5344, "S4ACS_GUI in"=w5363) -> ("error out"=w5380:errorcluster, "S4ACS_GUI out"=w5381:refnum<class "S4GUI.lvclass">)  [unwired: 7 in]
              }
              frame #3 {
                # "object"
                # "suffix"
                # "obsType"
                n2596 = call-dynamic "Read AcquisitionD.vi"("error in (no error)"=w5433, "S4ACS_GUI in"=w5434) -> ("error out"=w5424:errorcluster, "Acquisition.lvclass"=w5423:refnum<class "Acquisition.lvclass">, "S4ACS_GUI out"=w5414:refnum<class "S4GUI.lvclass">)  [unwired: 7 in]
                n2597 = local read "Exptime ch4"() -> (w5398:dbl)
                n2598 = call-dynamic "Read Channel.vi"("error in (no error)"=w5424, "Acquisition in"=w5423) -> ("error out"=w5421:errorcluster, "Channel.lvclass"=w5422:refnum<class "Channel.lvclass">, "Acquisition out"=w5413:refnum<class "Acquisition.lvclass">)  [unwired: 7 in]
                n2599 = call-dynamic "Read Interface.vi"("error in (no error)"=w5421, "Channel in"=w5422) -> ("error out"=w5429:errorcluster, "Interface.lvclass"=w5419:refnum<class "Interface.lvclass">, "Channel out"=w5420:refnum<class "Channel.lvclass">)  [unwired: 7 in]
                n2600 = call "Write Exposure Time.vi"("error in (no error)"=w5429, "Exposure Time"=w5398, "Interface in"=w5419) -> ("error out"=w5400:errorcluster, "Interface out"=w5402:refnum<class "Interface.lvclass">)  [unwired: 7 in]
                n2601 = case shown="Default" w5397 {
                  tunnel: w5402 -> [w5436 w5441]
                  tunnel: [w5436 w5440] -> w5401
                  tunnel: [w5435 w5439] -> w5399
                  tunnel: w5400 -> [w5435 w5438]
                  tunnel: w5398 -> [_ w5437]
                  frame "ZERO" {
                  }
                  frame Default {
                    n2602 = call-dynamic "Write prev ExpTime.vi"("error in (no error)"=w5438, "prev ExpTime"=w5437, "Interface in"=w5441) -> ("error out"=w5439:errorcluster, "Interface out"=w5440:refnum<class "Interface.lvclass">)  [unwired: 7 in]
                  }
                }
                n2603 = call-dynamic "Write Suffix.vi"("error in (no error)"=w5399, "Suffix"=w5430, "Interface in"=w5401) -> ("error out"=w5428:errorcluster, "Interface out"=w5418:refnum<class "Interface.lvclass">)  [unwired: 7 in]
                n2604 = call-dynamic "Write ObsType.vi"("error in (no error)"=w5428, "ObsType"=w5409, "Interface in"=w5418) -> ("error out"=w5427:errorcluster, "Interface out"=w5417:refnum<class "Interface.lvclass">)  [unwired: 7 in]
                n2605 = call-dynamic "Write Object.vi"("error in (no error)"=w5427, "Object"=w5408, "Interface in"=w5417) -> ("error out"=w5426:errorcluster, "Interface out"=w5416:refnum<class "Interface.lvclass">)  [unwired: 7 in]
                n2606 = call-dynamic "Write Comments.vi"("error in (no error)"=w5426, "Comments"=w5410, "Interface in"=w5416) -> ("error out"=w5425:errorcluster, "Interface out"=w5415:refnum<class "Interface.lvclass">)  [unwired: 7 in]
                n2607 = call-dynamic "Write DS9.vi"("error in (no error)"=w5425, "DS9"="F", "Interface in"=w5415) -> ("error out"=w5406:errorcluster, "Interface out"=w5407:refnum<class "Interface.lvclass">)  [unwired: 7 in]
                n2608 = property on="Exposure Time ch4" class="Slide (strict)"("Scale.Maximum"=w5398, "Scale.Minimum"=0.0 ("Scale.Range:Minimum")) -> ()  [unwired: 2 in, 2 out]
                n2609 = call-dynamic "Write Observer.vi"("error in (no error)"=w5406, "Observer"=w5405, "Interface in"=w5407) -> ("error out"=w5391:errorcluster, "Interface out"=w5392:refnum<class "Interface.lvclass">)  [unwired: 7 in]
                n2610 = call-dynamic "Write Interface.vi"("error in (no error)"=w5391, "Interface.lvclass"=w5392, "Channel in"=w5420) -> ("error out"=w5404:errorcluster, "Channel out"=w5403:refnum<class "Channel.lvclass">)  [unwired: 7 in]
                n2611 = call-dynamic "Write Channel.vi"("error in (no error)"=w5404, "Channel.lvclass"=w5403, "Acquisition in"=w5413) -> ("error out"=w5394:errorcluster, "Acquisition out"=w5396:refnum<class "Acquisition.lvclass">)  [unwired: 7 in]
                n2612 = call-dynamic "CalcCubeDuration.vi"("error in (no error)"=w5394, "Acquisition in"=w5396) -> ("error out"=w5393:errorcluster, "Acquisition out"=w5395:refnum<class "Acquisition.lvclass">)  [unwired: 8 in]
                n2613 = call-dynamic "Write AcquisitionD.vi"("error in (no error)"=w5393, "Acquisition.lvclass"=w5395, "S4ACS_GUI in"=w5414) -> ("error out"=w5431:errorcluster, "S4ACS_GUI out"=w5432:refnum<class "S4GUI.lvclass">)  [unwired: 7 in]
              }
            }
          }
        }
        n2614 = call-dynamic "Write User Event.vi"("error in (no error)"=w5041, "User Event"=w5038, "S4GUI in"=w5042) -> ("error out"=w5040:errorcluster, "S4GUI out"=w5039:refnum<class "S4GUI.lvclass">)  [unwired: 7 in]
        n2615 = property on="Pause SM" class="Bool"(error in=w5040, "DisabledEnum"=T12."Enabled" ("Disabled")) -> (error out=w5059:errorcluster)  [unwired: 1 in, 1 out]
      }
      event "# Cycles": Value Change {
        w5506 = 0.0 ("Scale.Range:Minor Increment")
        n2616 = event-data() -> ("NewVal"=w5442:u32)  [unwired: 1 in]
        n2617 = call-dynamic "Write ciclos.vi"("error in (no error)"=w5463, "ciclos"=w5442, "S4ACS_GUI in"=w5507) -> ("error out"=w5460:errorcluster, "S4ACS_GUI out"=w5462:refnum<class "S4GUI.lvclass">)  [unwired: 7 in]
        n2618 = call-dynamic "Write prev ciclos.vi"("error in (no error)"=w5460, "prev ciclos"=w5442, "S4GUI in"=w5462) -> ("error out"=w5459:errorcluster, "S4GUI out"=w5461:refnum<class "S4GUI.lvclass">)  [unwired: 7 in]
        n2619 = property on="#Cycles Done" class="Slide (strict)"("Scale.Maximum"=w5442, "Scale.Minimum"=w5506) -> ()  [unwired: 2 in, 2 out]
        n2620 = property on="Cycles Done ch2" class="Slide (strict)"("Scale.Maximum"=w5442, "Scale.Minimum"=w5506) -> ()  [unwired: 2 in, 2 out]
        n2621 = property on="Cycles Done ch4" class="Slide (strict)"("Scale.Maximum"=w5442, "Scale.Minimum"=w5506) -> ()  [unwired: 2 in, 2 out]
        n2622 = property on="Cycles Done ch1" class="Slide (strict)"("Scale.Maximum"=w5442, "Scale.Minimum"=w5506) -> ()  [unwired: 2 in, 2 out]
        n2623 = property on="Cycles Done ch3" class="Slide (strict)"("Scale.Maximum"=w5442, "Scale.Minimum"=w5506) -> ()  [unwired: 2 in, 2 out]
        n2624 = call-dynamic "Write TotalCiclos.vi"("error in (no error)"=w5459, "TotalCiclos"=w5442, "S4GUI in"=w5461) -> ("error out"=w5464:errorcluster, "S4GUI out"=w5465:refnum<class "S4GUI.lvclass">)  [unwired: 7 in]
        n2625 = call-dynamic "Read AcquisitionA.vi"("error in (no error)"=w5464, "S4ACS_GUI in"=w5465) -> ("error out"=w5500:errorcluster, "Acquisition.lvclass"=w5504:refnum<class "Acquisition.lvclass">, "S4ACS_GUI out"=w5505:refnum<class "S4GUI.lvclass">)  [unwired: 7 in]
        n2626 = call-dynamic "Read Channel.vi"("error in (no error)"=w5500, "Acquisition in"=w5504) -> ("error out"=w5499:errorcluster, "Channel.lvclass"=w5501:refnum<class "Channel.lvclass">, "Acquisition out"=w5503:refnum<class "Acquisition.lvclass">)  [unwired: 7 in]
        n2627 = call-dynamic "Write ciclos.vi"("error in (no error)"=w5499, "ciclos"=w5442, "Channel in"=w5501) -> ("error out"=w5457:errorcluster, "Channel out"=w5458:refnum<class "Channel.lvclass">)  [unwired: 7 in]
        n2628 = call-dynamic "Write prev ciclos.vi"("error in (no error)"=w5457, "prev ciclos"=w5442, "Channel in"=w5458) -> ("error out"=w5456:errorcluster, "Channel out"=w5455:refnum<class "Channel.lvclass">)  [unwired: 7 in]
        n2629 = call-dynamic "Write Channel.vi"("error in (no error)"=w5456, "Channel.lvclass"=w5455, "Acquisition in"=w5503) -> ("error out"=w5498:errorcluster, "Acquisition out"=w5502:refnum<class "Acquisition.lvclass">)  [unwired: 7 in]
        n2630 = call-dynamic "Write AcquisitionA.vi"("error in (no error)"=w5498, "Acquisition.lvclass"=w5502, "S4ACS_GUI in"=w5505) -> ("error out"=w5490:errorcluster, "S4ACS_GUI out"=w5495:refnum<class "S4GUI.lvclass">)  [unwired: 7 in]
        n2631 = call "Read AcquisitionB.vi"("error in (no error)"=w5490, "S4ACS_GUI in"=w5495) -> ("error out"=w5489:errorcluster, "Acquisition.lvclass"=w5493:refnum<class "Acquisition.lvclass">, "S4ACS_GUI out"=w5494:refnum<class "S4GUI.lvclass">)  [unwired: 7 in]
        n2632 = call-dynamic "Read Channel.vi"("error in (no error)"=w5489, "Acquisition in"=w5493) -> ("error out"=w5496:errorcluster, "Channel.lvclass"=w5497:refnum<class "Channel.lvclass">, "Acquisition out"=w5492:refnum<class "Acquisition.lvclass">)  [unwired: 7 in]
        n2633 = call-dynamic "Write ciclos.vi"("error in (no error)"=w5496, "ciclos"=w5442, "Channel in"=w5497) -> ("error out"=w5454:errorcluster, "Channel out"=w5453:refnum<class "Channel.lvclass">)  [unwired: 7 in]
        n2634 = call-dynamic "Write prev ciclos.vi"("error in (no error)"=w5454, "prev ciclos"=w5442, "Channel in"=w5453) -> ("error out"=w5451:errorcluster, "Channel out"=w5452:refnum<class "Channel.lvclass">)  [unwired: 7 in]
        n2635 = call-dynamic "Write Channel.vi"("error in (no error)"=w5451, "Channel.lvclass"=w5452, "Acquisition in"=w5492) -> ("error out"=w5488:errorcluster, "Acquisition out"=w5491:refnum<class "Acquisition.lvclass">)  [unwired: 7 in]
        n2636 = call "Write AcquisitionB.vi"("error in (no error)"=w5488, "Acquisition.lvclass"=w5491, "S4ACS_GUI in"=w5494) -> ("error out"=w5483:errorcluster, "S4ACS_GUI out"=w5484:refnum<class "S4GUI.lvclass">)  [unwired: 7 in]
        n2637 = call-dynamic "Read AcquisitionC.vi"("error in (no error)"=w5483, "S4ACS_GUI in"=w5484) -> ("error out"=w5480:errorcluster, "Acquisition.lvclass"=w5481:refnum<class "Acquisition.lvclass">, "S4ACS_GUI out"=w5482:refnum<class "S4GUI.lvclass">)  [unwired: 7 in]
        n2638 = call-dynamic "Read Channel.vi"("error in (no error)"=w5480, "Acquisition in"=w5481) -> ("error out"=w5486:errorcluster, "Channel.lvclass"=w5487:refnum<class "Channel.lvclass">, "Acquisition out"=w5485:refnum<class "Acquisition.lvclass">)  [unwired: 7 in]
        n2639 = call-dynamic "Write ciclos.vi"("error in (no error)"=w5486, "ciclos"=w5442, "Channel in"=w5487) -> ("error out"=w5449:errorcluster, "Channel out"=w5450:refnum<class "Channel.lvclass">)  [unwired: 7 in]
        n2640 = call-dynamic "Write prev ciclos.vi"("error in (no error)"=w5449, "prev ciclos"=w5442, "Channel in"=w5450) -> ("error out"=w5448:errorcluster, "Channel out"=w5447:refnum<class "Channel.lvclass">)  [unwired: 7 in]
        n2641 = call-dynamic "Write Channel.vi"("error in (no error)"=w5448, "Channel.lvclass"=w5447, "Acquisition in"=w5485) -> ("error out"=w5478:errorcluster, "Acquisition out"=w5479:refnum<class "Acquisition.lvclass">)  [unwired: 7 in]
        n2642 = call-dynamic "Write AcquisitionC.vi"("error in (no error)"=w5478, "Acquisition.lvclass"=w5479, "S4ACS_GUI in"=w5482) -> ("error out"=w5472:errorcluster, "S4ACS_GUI out"=w5473:refnum<class "S4GUI.lvclass">)  [unwired: 7 in]
        n2643 = call-dynamic "Read AcquisitionD.vi"("error in (no error)"=w5472, "S4ACS_GUI in"=w5473) -> ("error out"=w5471:errorcluster, "Acquisition.lvclass"=w5470:refnum<class "Acquisition.lvclass">, "S4ACS_GUI out"=w5474:refnum<class "S4GUI.lvclass">)  [unwired: 7 in]
        n2644 = call-dynamic "Read Channel.vi"("error in (no error)"=w5471, "Acquisition in"=w5470) -> ("error out"=w5476:errorcluster, "Channel.lvclass"=w5477:refnum<class "Channel.lvclass">, "Acquisition out"=w5475:refnum<class "Acquisition.lvclass">)  [unwired: 7 in]
        n2645 = call-dynamic "Write ciclos.vi"("error in (no error)"=w5476, "ciclos"=w5442, "Channel in"=w5477) -> ("error out"=w5445:errorcluster, "Channel out"=w5446:refnum<class "Channel.lvclass">)  [unwired: 7 in]
        n2646 = call-dynamic "Write prev ciclos.vi"("error in (no error)"=w5445, "prev ciclos"=w5442, "Channel in"=w5446) -> ("error out"=w5444:errorcluster, "Channel out"=w5443:refnum<class "Channel.lvclass">)  [unwired: 7 in]
        n2647 = call-dynamic "Write Channel.vi"("error in (no error)"=w5444, "Channel.lvclass"=w5443, "Acquisition in"=w5475) -> ("error out"=w5469:errorcluster, "Acquisition out"=w5468:refnum<class "Acquisition.lvclass">)  [unwired: 7 in]
        n2648 = call-dynamic "Write AcquisitionD.vi"("error in (no error)"=w5469, "Acquisition.lvclass"=w5468, "S4ACS_GUI in"=w5474) -> ("error out"=w5466:errorcluster, "S4ACS_GUI out"=w5467:refnum<class "S4GUI.lvclass">)  [unwired: 7 in]
      }
      event "AllConfig": Value Change {
        n2649 = event-data() -> ()  [unwired: 1 in, 6 out]
        n2650 = call "Read Instrument.lvclass.vi"("error in (no error)"=w5512, "S4ACS_GUI in"=w5513) -> ("error out"=w5592:errorcluster, "Instrument.lvclass"=w5559:refnum<class "Instrument.lvclass">, "S4ACS_GUI out"=w5590:refnum<class "S4GUI.lvclass">)  [unwired: 7 in]
        n2651 = call "Read ASEL.vi"("error in (no error)"=w5592, "Instrument in"=w5559) -> ("error out"=w5584:errorcluster, "Opt_Selector.lvclass"=w5583:refnum<class "Opt_Selector.lvclass">, "Instrument out"=w5591:refnum<class "Instrument.lvclass">)  [unwired: 7 in]
        n2652 = call-dynamic "Read State Machine.vi"("error in (no error)"=w5584, "Device in"=w5583) -> ("error out"=w5587:errorcluster, "State Machine.lvclass"=w5589:refnum<class "State Machine.lvclass">, "Device out"=w5581:refnum<class "Opt_Selector.lvclass">)  [unwired: 7 in]
        n2653 = call "Next State.vi"("error in (no error)"=w5587, "New_State"=1, "State Machine in"=w5589) -> ("error out"=w5586:errorcluster, "State Machine out"=w5585:refnum<class "State Machine.lvclass">)  [unwired: 7 in]
        n2654 = call-dynamic "Write State Machine.vi"("error in (no error)"=w5586, "State Machine.lvclass"=w5585, "Device in"=w5581) -> ("error out"=w5580:errorcluster, "Device out"=w5582:refnum<class "Opt_Selector.lvclass">)  [unwired: 7 in]
